vi "Experiment_parameters.vi"() -> ()   [LabVIEW 2016]
panel:
  in  "Experiment parameters":T1={"Stimulus signal"={"Effector"="On-screen signal", "Delay"=-100.0}, "Reward period signal"={"Effector"="On-screen signal", "Delay"=0.0}, "Reward"={"Effector"="On-screen signal", "Condition"="In window", "Delay"=100.0}, "Response"={"Source"="Keyboard", "Window start"=0.0, "Threshold"=1, "Window duration"=250.0}, "Punishment"={"Effector"="On-screen signal", "Condition"="Wrong response"}}
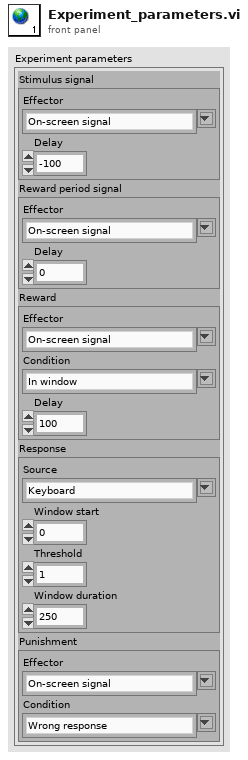
[diagram p1: front panel]
types:
  T1 = cluster{"Stimulus signal":cluster{"Effector":string, "Delay":dbl}, "Reward period signal":cluster{"Effector":string, "Delay":dbl}, "Reward":cluster{"Effector":string, "Condition":string, "Delay":dbl}, "Response":cluster{"Source":string, "Window start":dbl, "Threshold":u32, "Window duration":dbl}, "Punishment":cluster{"Effector":string, "Condition":string}}
diagram:
